vi "output_on_PSG.vi"(5 "Enable RF Output (F:Disable)":bool) -> ()   [LabVIEW 2011]
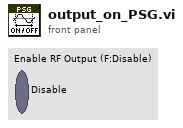
[diagram p1: front panel]
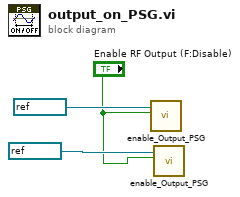
[diagram p0: block diagram]
diagram:
  n1 = call "enable_Output_PSG.vi"("Enable RF Output (F:Disable)"="Enable RF Output (F:Disable)", "VISA resource name"=refnum<visa-resource-name> "PSG1" ("VISA resource name 2")) -> ()  [unwired: 8 in, 2 out]
  n2 = call "enable_Output_PSG.vi"("Enable RF Output (F:Disable)"="Enable RF Output (F:Disable)", "VISA resource name"=refnum<visa-resource-name> "PSG2" ("VISA resource name 2")) -> ()  [unwired: 8 in, 2 out]
